vi "Update.vi"(8 "error in (no error)":errorcluster, 10 "Message in":refnum<class "UpdateMessage.lvclass">, 11 "Tomo in":refnum<class "Tomo.lvclass">) -> (0 "error out":errorcluster, 3 "Tomo out":refnum<class "Tomo.lvclass">)   [LabVIEW 2012, in "Tomo.lvclass"]
doc: "The update method processes the command 'update'. \n\nThe command 'update' is used for receiving new values to be set to the private data of the class. This could be seen as a public set method for setting new parameters to the private class data."
uses:
  Tomo.lvclass
  <vilib>/Distrio/Murmex/Murmex/Murmex.lvclass
  <vilib>/Distrio/Murmex/UpdateMessage/UpdateMessage.lvclass
  <vilib>/Distrio/Murmex/GenericMessage/GenericMessage.lvclass
panel:
  # "This method is called when the UPDATE\ntrigger is sent. \n\nOverride this method when your component needs to\nrespond to this trigger. \n\nCall parent for proper implementation"
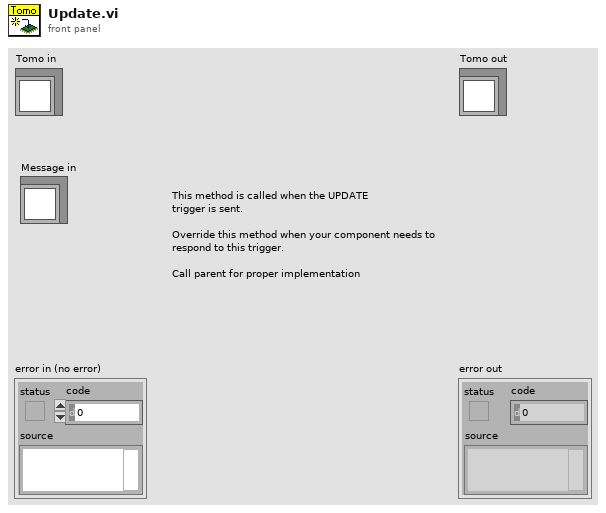
[diagram p1: front panel]
types:
  T1 = enum16{"Cubic volume", "Custom volume", "Self-generate volume"}
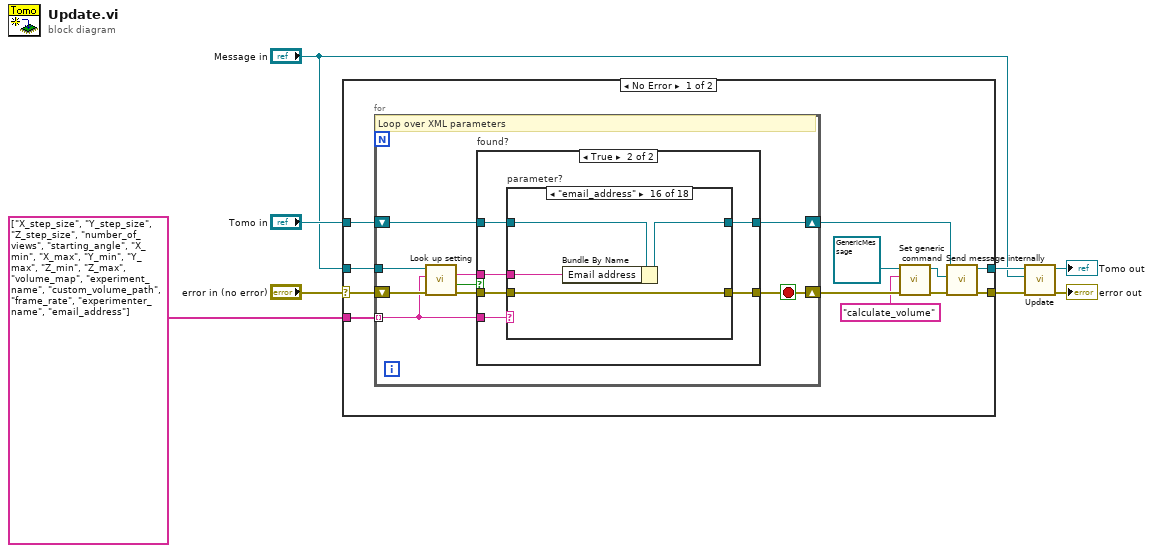
[diagram p0: block diagram]
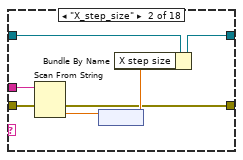
[diagram p4: hidden frame]
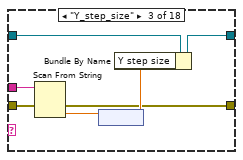
[diagram p5: hidden frame]
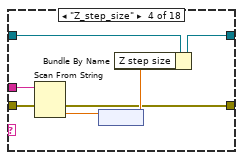
[diagram p6: hidden frame]
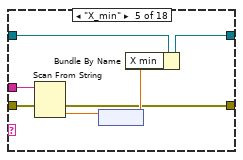
[diagram p7: hidden frame]
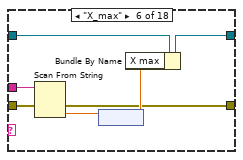
[diagram p8: hidden frame]
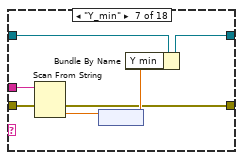
[diagram p9: hidden frame]
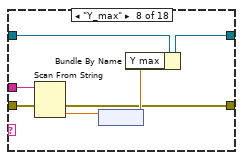
[diagram p10: hidden frame]
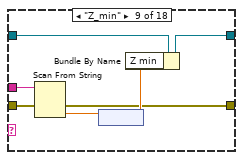
[diagram p11: hidden frame]
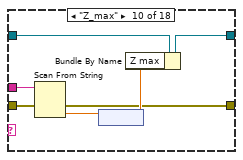
[diagram p12: hidden frame]
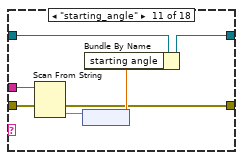
[diagram p13: hidden frame]
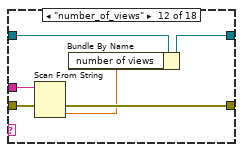
[diagram p14: hidden frame]
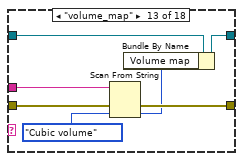
[diagram p15: hidden frame]
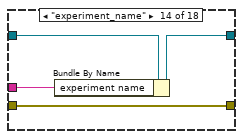
[diagram p16: hidden frame]
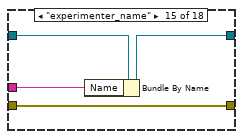
[diagram p17: hidden frame]
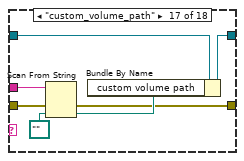
[diagram p18: hidden frame]
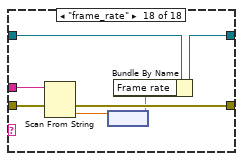
[diagram p19: hidden frame]
diagram:
  n1 = case shown="No Error" "error in (no error)" {
    selector: "error in (no error)" -> [w20 w149]
    tunnel: "Message in" -> [w19 _]
    tunnel: "Tomo in" -> [w18 w150]
    tunnel: string[] ["X_step_size", "Y_step_size", "Z_step_size", "number_of_views", "starting_angle", "X_min", "X_max", "Y_min", "Y_max", "Z_min", "Z_max", "volume_map", "experiment_name", "custom_volume_path", "frame_rate", "experimenter_name", "email_address"] -> [w17 _]
    tunnel: [w15 w149] -> w3
    tunnel: [w12 w150] -> w2
    frame No Error {
      n2 = for {
        shift-right: [w22] -> w16
        shift-left: w20 -> [w29]
        tunnel: w19 -> [w28]
        shift-right: [w23] -> w13
        shift-left: w18 -> [w24]
        tunnel: w17 -> [w21] mode=indexing
        stop <- w22 stop-if-true
        # "Loop over XML parameters"
        n3 = call <vilib>:"Look up setting.vi"("error in (no error)"=w29, "tag name"=w21, "UpdateMessage in"=w28) -> ("error out"=w26:errorcluster, "found?"=w27:bool, "value"=w25:string)  [unwired: 5 in, 1 out]
        n4 = case "found?" shown="True" w27 {
          tunnel: w21 -> [_ w37]
          tunnel: w26 -> [w30 w35]
          tunnel: w25 -> [_ w34]
          tunnel: w24 -> [w31 w36]
          tunnel: [w30 w33] -> w22
          tunnel: [w31 w32] -> w23
          frame False {
          }
          frame True {
            n5 = case "parameter?" shown="\"email_address\"" w37 {
              tunnel: w36 -> [w39 w44 w51 w58 w65 w72 w79 w86 w93 w100 w107 w113 w120 w126 w130 w134 w141 w148]
              tunnel: w35 -> [w38 w46 w53 w60 w67 w74 w81 w88 w95 w102 w109 w115 w122 w124 w128 w132 w135 w143]
              tunnel: w34 -> [_ w45 w52 w59 w66 w73 w80 w87 w94 w101 w108 w114 w121 w123 w127 w131 w139 w146]
              tunnel: [w38 w41 w48 w55 w62 w69 w76 w83 w90 w97 w104 w112 w119 w124 w128 w132 w136 w144] -> w33
              tunnel: [w39 w40 w47 w54 w61 w68 w75 w82 w89 w96 w103 w111 w118 w125 w129 w133 w140 w147] -> w32
              frame Default {
              }
              frame "X_step_size" {
                n6 = Scan From String(input string=w45, error in=w46) -> (error out=w41:errorcluster, output 1=w42:dbl)  [unwired: 3 in, 2 out]
                n7 = node(w42) -> (w43:dbl[unit])
                n8 = Bundle By Name(cluster=w44, "X step size"=w43) -> (w40:refnum<class "Tomo.lvclass">)
              }
              frame "Y_step_size" {
                n9 = Scan From String(input string=w52, error in=w53) -> (error out=w48:errorcluster, output 1=w49:dbl)  [unwired: 3 in, 2 out]
                n10 = node(w49) -> (w50:dbl[unit])
                n11 = Bundle By Name(cluster=w51, "Y step size"=w50) -> (w47:refnum<class "Tomo.lvclass">)
              }
              frame "Z_step_size" {
                n12 = Scan From String(input string=w59, error in=w60) -> (error out=w55:errorcluster, output 1=w56:dbl)  [unwired: 3 in, 2 out]
                n13 = node(w56) -> (w57:dbl[unit])
                n14 = Bundle By Name(cluster=w58, "Z step size"=w57) -> (w54:refnum<class "Tomo.lvclass">)
              }
              frame "X_min" {
                n15 = Scan From String(input string=w66, error in=w67) -> (error out=w62:errorcluster, output 1=w63:dbl)  [unwired: 3 in, 2 out]
                n16 = node(w63) -> (w64:dbl[unit])
                n17 = Bundle By Name(cluster=w65, "X min"=w64) -> (w61:refnum<class "Tomo.lvclass">)
              }
              frame "X_max" {
                n18 = Scan From String(input string=w73, error in=w74) -> (error out=w69:errorcluster, output 1=w70:dbl)  [unwired: 3 in, 2 out]
                n19 = node(w70) -> (w71:dbl[unit])
                n20 = Bundle By Name(cluster=w72, "X max"=w71) -> (w68:refnum<class "Tomo.lvclass">)
              }
              frame "Y_min" {
                n21 = Scan From String(input string=w80, error in=w81) -> (error out=w76:errorcluster, output 1=w77:dbl)  [unwired: 3 in, 2 out]
                n22 = node(w77) -> (w78:dbl[unit])
                n23 = Bundle By Name(cluster=w79, "Y min"=w78) -> (w75:refnum<class "Tomo.lvclass">)
              }
              frame "Y_max" {
                n24 = Scan From String(input string=w87, error in=w88) -> (error out=w83:errorcluster, output 1=w84:dbl)  [unwired: 3 in, 2 out]
                n25 = node(w84) -> (w85:dbl[unit])
                n26 = Bundle By Name(cluster=w86, "Y max"=w85) -> (w82:refnum<class "Tomo.lvclass">)
              }
              frame "Z_min" {
                n27 = Scan From String(input string=w94, error in=w95) -> (error out=w90:errorcluster, output 1=w91:dbl)  [unwired: 3 in, 2 out]
                n28 = node(w91) -> (w92:dbl[unit])
                n29 = Bundle By Name(cluster=w93, "Z min"=w92) -> (w89:refnum<class "Tomo.lvclass">)
              }
              frame "Z_max" {
                n30 = Scan From String(input string=w101, error in=w102) -> (error out=w97:errorcluster, output 1=w98:dbl)  [unwired: 3 in, 2 out]
                n31 = node(w98) -> (w99:dbl[unit])
                n32 = Bundle By Name(cluster=w100, "Z max"=w99) -> (w96:refnum<class "Tomo.lvclass">)
              }
              frame "starting_angle" {
                n33 = Scan From String(input string=w108, error in=w109) -> (error out=w104:errorcluster, output 1=w105:dbl)  [unwired: 3 in, 2 out]
                n34 = node(w105) -> (w106:dbl[unit])
                n35 = Bundle By Name(cluster=w107, "starting angle"=w106) -> (w103:refnum<class "Tomo.lvclass">)
              }
              frame "number_of_views" {
                n36 = Scan From String(input string=w114, error in=w115) -> (error out=w112:errorcluster, output 1=w110:dbl)  [unwired: 3 in, 2 out]
                n37 = Bundle By Name(cluster=w113, "number of views"=w110) -> (w111:refnum<class "Tomo.lvclass">)
              }
              frame "volume_map" {
                n38 = Scan From String(input string=w121, error in=w122, default 1=T1."Cubic volume" ("Volume map")) -> (error out=w119:errorcluster, output 1=w116:T1)  [unwired: 2 in, 2 out]
                n39 = Bundle By Name(cluster=w120, "Volume map"=w116) -> (w118:refnum<class "Tomo.lvclass">)
              }
              frame "experiment_name" {
                n40 = Bundle By Name(cluster=w126, "experiment name"=w123) -> (w125:refnum<class "Tomo.lvclass">)
              }
              frame "experimenter_name" {
                n41 = Bundle By Name(cluster=w130, "Name"=w127) -> (w129:refnum<class "Tomo.lvclass">)
              }
              frame "email_address" {
                n42 = Bundle By Name(cluster=w134, "Email address"=w131) -> (w133:refnum<class "Tomo.lvclass">)
              }
              frame "custom_volume_path" {
                n43 = Scan From String(input string=w139, error in=w135, default 1=path "") -> (error out=w136:errorcluster, output 1=w137:path)  [unwired: 2 in, 2 out]
                n44 = Bundle By Name(cluster=w141, "custom volume path"=w137) -> (w140:refnum<class "Tomo.lvclass">)
              }
              frame "frame_rate" {
                n45 = Scan From String(input string=w146, error in=w143) -> (error out=w144:errorcluster, output 1=w145:dbl)  [unwired: 3 in, 2 out]
                n46 = node(w145) -> (w142:dbl[unit])
                n47 = Bundle By Name(cluster=w148, "Frame rate"=w142) -> (w147:refnum<class "Tomo.lvclass">)
              }
            }
          }
        }
      }
      n48 = call <vilib>:"Set generic command.vi"("error in (no error)"=w16, "generic command"="calculate_volume", "GenericMessage in"=refnum<class "GenericMessage.lvclass"> refnum) -> ("error out"=w14:errorcluster, "GenericMessage out"=w11:refnum<class "GenericMessage.lvclass">)  [unwired: 7 in]
      n49 = call <vilib>:"Send message internally.vi"("error in (no error)"=w14, "Message"=w11, "Murmex in"=w13) -> ("error out"=w15:errorcluster, "Murmex out"=w12:refnum<class "Tomo.lvclass">)  [unwired: 7 in]
    }
    frame Error {
    }
  }
  n50 = call-parent "Update.vi"("error in (no error)"=w3, "Message in"="Message in", "Murmex in"=w2) -> ("error out"=→"error out":errorcluster, "Murmex out"=→"Tomo out":refnum<class "Tomo.lvclass">)  [unwired: 7 in]
